vi "氨氮总磷质控流程.vi"(0 "队列输入":refnum<queue>, 5 "氨氮":bool, 7 "氨氮量程切换":enum32{"H", "L", "AUTO"}(ring)=enum."AUTO", 9 "总磷":bool, 11 "总磷量程切换":enum32{"H", "L", "AUTO"}(ring)=enum."AUTO") -> (4 "布尔":bool, 6 "总磷中断报警":bool, 8 "氨氮中断报警":bool)   [LabVIEW 2016]
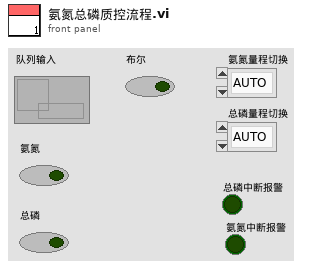
[diagram p1: front panel]
types:
  T1 = enum16{"待机", "启动氨氮水样", "氨氮测量中", "启动氨氮加标", "启动氨氮加标回收", "氨氮加标回收测量中", "启动总磷水样", "总磷水样测量中", "启动总磷加标", "启动总磷加标回收", "总磷加标回收测量中", "结束"}
  T2 = cluster{"站号":u16, "量程切换":enum32{"H", "L", "AUTO"}, "控制命令":enum16{"启动测量", "标样核查", "零点核查", "跨度核查", "空白测试", "平行样测试", "加标回收", "空白校准", "标样校准", "初始化（清洗）", "停止测试", "仪器重启", "校时", "模式设置", "测量间隔设置", "盲样测试"}, "模式设置":enum16{"待机", "连续模式", "周期模式", "定点模式", "受控模式", "手动模式"}, "测量间隔":u16}
  T3 = cluster{"时间标识":timestamp, "设备":string, "日志信息":string}
  T4 = cluster{"系统时间":timestamp, "工作状态":enum16{"空闲", "水样测试", "标样核查", "零点核查", "跨度核查", "空白测试", "平行样测试", "加标回收", "空白校准", "标样校准", "初始化（清洗）"}, "测量模式":enum16{"待机", "连续模式", "周期模式", "定点模式", "受控模式", "手动模式"}, "告警代码":enum16{"无告警", "缺试剂告警", "缺水样告警", "缺蒸馏水告警", "缺标液告警", "仪表漏液告警", "标定异常告警", "超量程告警", "加热异常", "低试剂预警", "超上限告警", "超下限告警", "仪表内部其他异常", "滴定异常告警", "电极异常告警", "量程切换告警", "参数设置告警", "PH电极电位异常", "电导率电极异常", "浊度光度异常", "溶解氧电极异常", "溶解氧光强异常", "温度异常告警", "PH异常告警", "溶解氧异常告警", "电导率异常告警", "浊度异常告警", "叶绿素异常告警", "藻密度异常告警", "蓝绿藻异常告警", "ORP异常告警", "氨氮异常告警", "清洁刷异常告警", "SD卡异常告警", "蓝牙异常告警", "Wifi异常告警", "流程异常告警"}, "故障代码":enum16{"无故障", "电机故障", "温度故障", "通讯故障", "滴定故障"}, "日志代码":u16, "软件版本":u16, "F0":sgl, "F1":sgl, "F2":sgl, "F3":sgl, "T":sgl, "H":sgl, "id":u16, "flowid":u16, "量程":u16, "总磷控温温度1":sgl, "营养盐控温温度2":sgl, "ADC":sgl}
  T5 = enum16{"空闲", "水样测试", "标样核查", "零点核查", "跨度核查", "空白测试", "平行样测试", "加标回收", "空白校准", "标样校准", "初始化（清洗）"}
  T6 = cluster{"因子编码":u32, "单位":u16, "标样参考值":sgl, "水样数据时间":timestamp, "水样实测值":sgl, "水样数据标识":string, "标样数据时间":timestamp, "标样实测值":sgl, "标样数据标识":string, "空白数据时间":timestamp, "空白实测值":sgl, "空白数据标识":string, "零点核查数据时间":timestamp, "零点核查实测值":sgl, "零点核查数据标识":string, "跨度核查数据时间":timestamp, "跨度核查实测值":sgl, "跨度核查数据标识":string, "加标回收数据时间":timestamp, "加标回收实测值":sgl, "加标回收数据标识":string, "平行样数据时间":timestamp, "平行样实测值":sgl, "平行样数据标识":string}
  T7 = cluster{"量程":dbl, "检出限":dbl, "加标前水样浓度":dbl, "加标后水样浓度":dbl, "加标水杯定容体积":dbl, "加标母液浓度":dbl, "加标体积":dbl, "加标回收率":dbl}
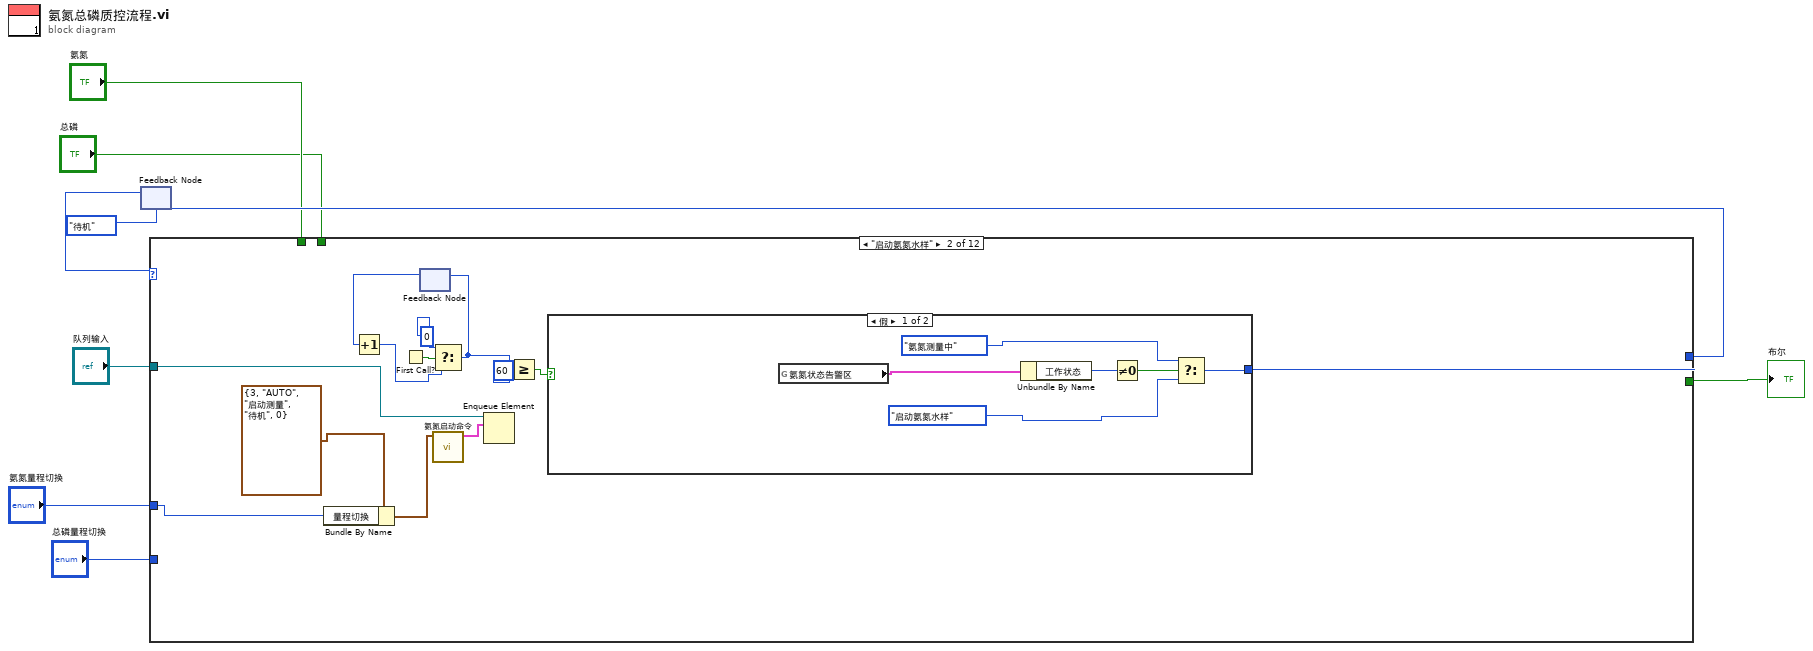
[diagram p0: block diagram]
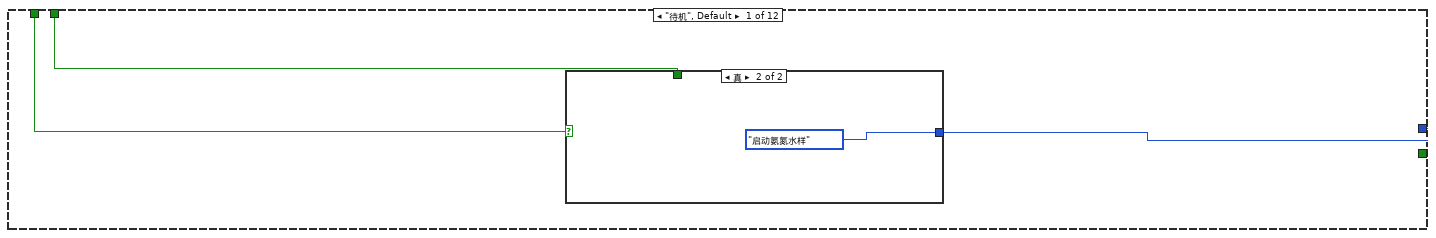
[diagram p2: hidden frame]
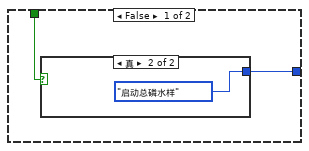
[diagram p3: hidden frame]
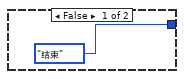
[diagram p4: hidden frame]
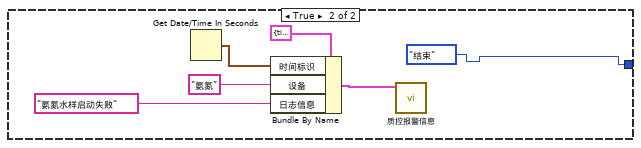
[diagram p5: hidden frame]
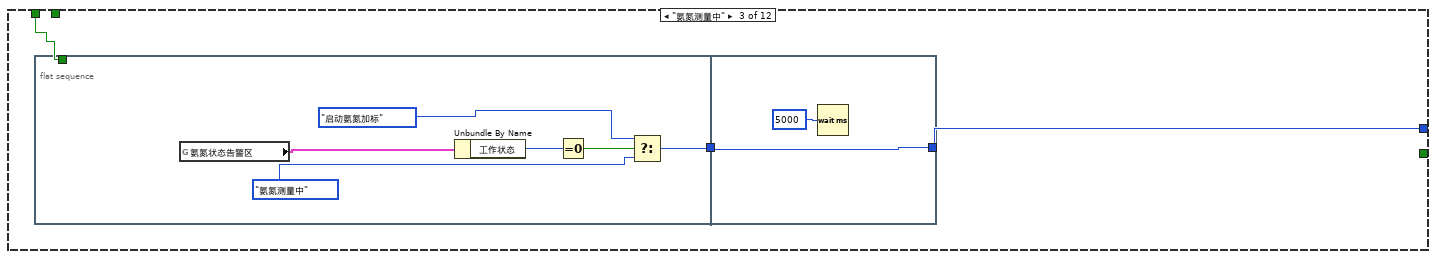
[diagram p6: hidden frame]
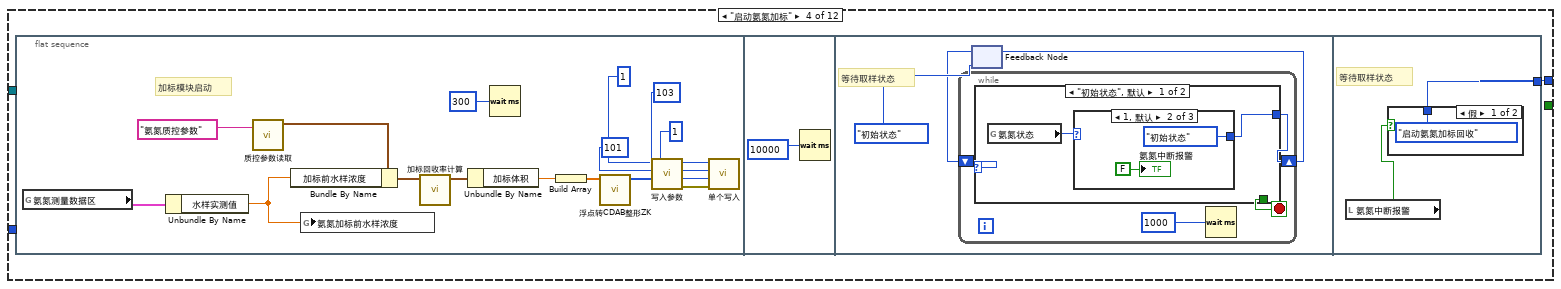
[diagram p7: hidden frame]
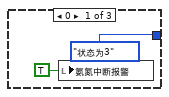
[diagram p8: hidden frame]
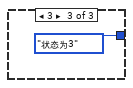
[diagram p9: hidden frame]
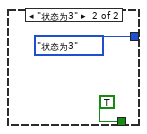
[diagram p10: hidden frame]
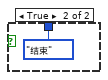
[diagram p11: hidden frame]
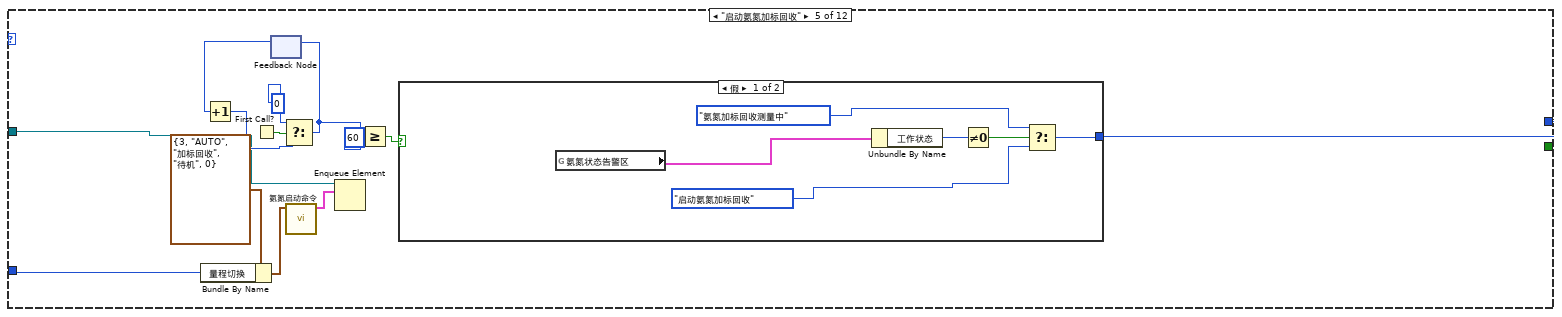
[diagram p12: hidden frame]
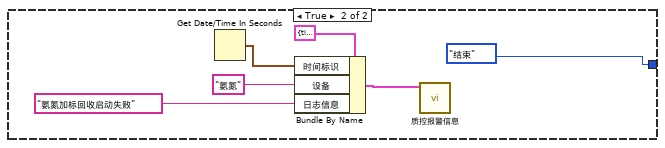
[diagram p13: hidden frame]
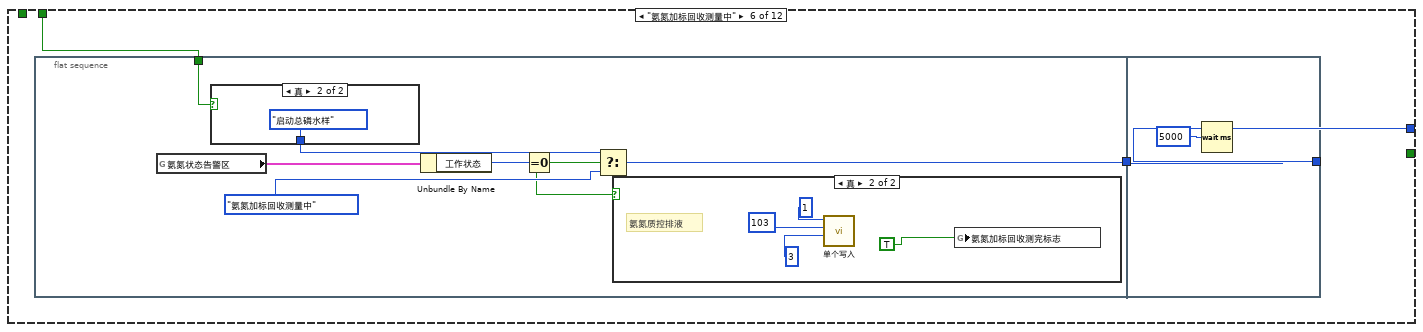
[diagram p14: hidden frame]
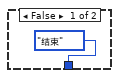
[diagram p15: hidden frame]
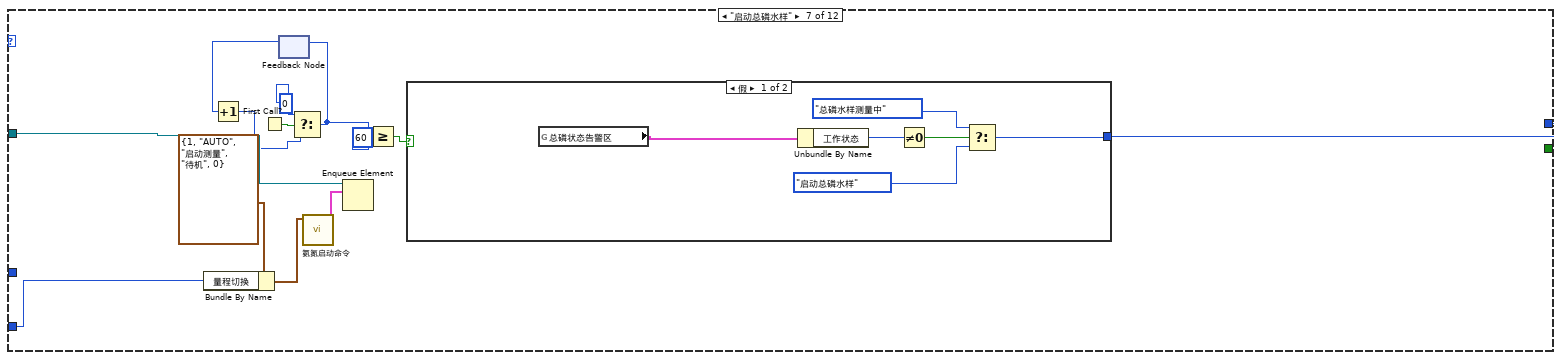
[diagram p17: hidden frame]
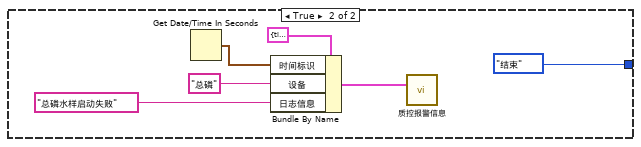
[diagram p18: hidden frame]
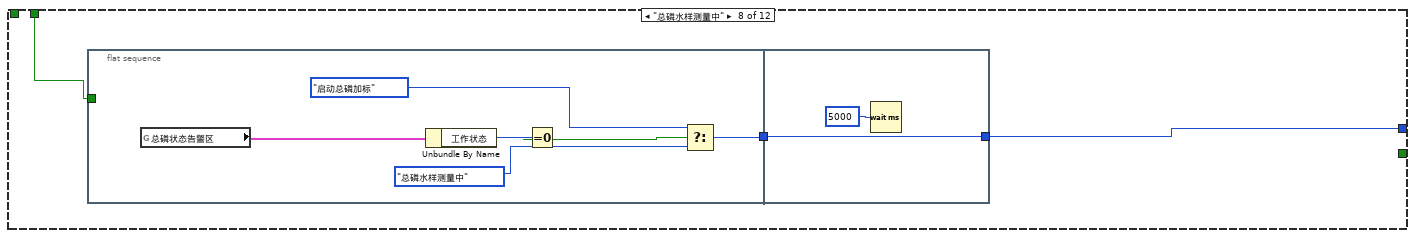
[diagram p19: hidden frame]
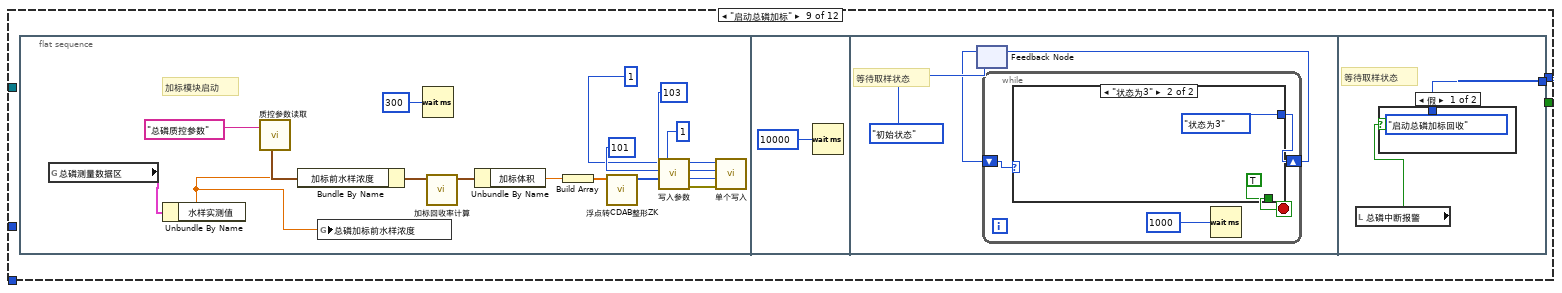
[diagram p20: hidden frame]
diagram:
  n1 = feedback #1(T1."待机") -> (w8:T1)
  n2 = case shown="\"启动氨氮水样\"" w8 {
    tunnel: [w12 w29 w45 w54 w95 w117 w145 w161 w170 w211 w232 T1."结束"] -> w7
    tunnel: "队列输入" -> [_ w30 _ _ w96 _ w146 _ _ w212 _ _]
    tunnel: [_ _ _ _ _ _ _ _ _ _ _ TRUE] -> w4
    tunnel: "总磷" -> [w10 _ _ _ _ w116 _ w159 _ _ _ _]
    tunnel: "氨氮" -> [w11 _ w43 _ _ _ _ _ _ _ _ _]
    tunnel: "氨氮量程切换" -> [_ w19 _ _ w92 _ _ _ _ _ _ _]
    tunnel: "总磷量程切换" -> [_ _ _ _ _ _ w134 _ _ w210 _ _]
    frame "待机", Default {
      n3 = case shown="真" w11 {
        tunnel: [w13 T1."启动氨氮水样"] -> w12
        tunnel: w10 -> [w14 _]
        frame False {
          n4 = case shown="真" w14 {
            tunnel: [T1."结束" T1."启动总磷水样"] -> w13
            frame False {
            }
            frame True {
            }
          }
        }
        frame True {
        }
      }
    }
    frame "启动氨氮水样" {
      n5 = Bundle By Name(cluster=T2 {"站号"=3, "量程切换"=enum."AUTO", "控制命令"=enum."启动测量", "模式设置"=enum."待机", "测量间隔"=0} ("参数"), "量程切换"=w19) -> (w18:T2)
      n6 = First Call?() -> (First Call?: T/F=w27:bool)
      n7 = feedback #2() -> (w26:i32)  [unwired: 1 in]
      n8 = Increment(x=w26) -> (x+1=w25:i32)
      n9 = Select(t=0, s=w27, f=w25) -> (s? t:f=w24:i32)
      n10 = feedback-in #2(w24) -> ()
      n11 = call "氨氮启动命令.vi"("参数"=w18) -> ("启动命令"=w21:cluster{"命令":string, "data":variant})  [unwired: 10 in]
      n12 = Enqueue Element(queue=w30, element=w21) -> ()  [unwired: 2 in, 3 out]
      n13 = Greater Or Equal?(x=w24, y=60) -> (x >= y?=w22:bool)
      n14 = case shown="假" w22 {
        tunnel: [w34 T1."结束"] -> w29
        frame False {
          n15 = global read "与氨氮交互全局.vi" "氨氮状态告警区"() -> (w31:T4)
          n16 = Unbundle By Name(w31) -> ("工作状态"=w36:T5)
          n17 = Not Equal To 0?(x=w36) -> (x != 0?=w35:bool)
          n18 = Select(t=T1."氨氮测量中", s=w35, f=T1."启动氨氮水样") -> (s? t:f=w34:T1)
        }
        frame True {
          n19 = Get Date/Time In Seconds() -> (seconds since 1Jan1904=w42:timestamp)
          n20 = Bundle By Name(cluster=T3 {"时间标识"=timestamp(0 s since 1904-01-01), "设备"="", "日志信息"=""} ("data in"), "时间标识"=w42, "设备"="氨氮", "日志信息"="氨氮水样启动失败") -> (w38:T3)
          n21 = call "质控报警信息.vi"("data in"=w38) -> ()  [unwired: 11 in]
        }
      }
    }
    frame "氨氮测量中" {
      n22 = flat-sequence {
        tunnel: [w50] -> w44
        tunnel: w43 -> [_]
        tunnel: [w53] -> w45
        tunnel: w44 -> [w53]
        frame #0 {
          n23 = global read "与氨氮交互全局.vi" "氨氮状态告警区"() -> (w46:T4)
          n24 = Unbundle By Name(w46) -> ("工作状态"=w51:T5)
          n25 = Equal To 0?(x=w51) -> (x = 0?=w49:bool)
          n26 = Select(t=T1."启动氨氮加标", s=w49, f=T1."氨氮测量中") -> (s? t:f=w50:T1)
        }
        frame #1 {
          n27 = Wait (ms)(milliseconds to wait=u32 5000 ("等待时间（毫秒）")) -> ()  [unwired: 1 out]
        }
      }
    }
    frame "启动氨氮加标" {
      n28 = flat-sequence {
        tunnel: [w88] -> w54
        frame #0 {
          w59 = u16 1 ("value")
          # "加标模块启动"
          n29 = global read "与氨氮交互全局.vi" "氨氮测量数据区"() -> (w56:T6)
          n30 = Unbundle By Name(w56) -> ("水样实测值"=w57:sgl)
          n31 = call "质控参数读取.vi"("section"="氨氮质控参数") -> ("参数"=w67:T7)  [unwired: 9 in, 1 out]
          n32 = Bundle By Name(cluster=w67, "加标前水样浓度"=w57) -> (w68:T7)
          n33 = global write "水样浓度全局.vi" "氨氮加标前水样浓度"(w57) -> ()
          n34 = call "加标回收率计算.vi"("参数"=w68) -> ("参数 out"=w66:T7)  [unwired: 10 in]
          n35 = Unbundle By Name(w66) -> ("加标体积"=w58:dbl)
          n36 = Wait (ms)(milliseconds to wait=u32 300 ("等待时间（毫秒）")) -> ()  [unwired: 1 out]
          n37 = Build Array(w58) -> (w65:dbl[])
          n38 = call "浮点转CDAB整形ZK.vi"("浮点数"=w65) -> ("CDAB整形输出"=w60:u16[])  [unwired: 10 in]
          n39 = call "写入参数.vi"("values"=w60, "starting address"=u16 101, "Slave ID"=w59) -> ("error out"=w64:errorcluster)  [unwired: 8 in]
          n40 = call "单个写入.vi"("Error in"=w64, "value"=u16 1, "address"=u16 103, "Slave ID"=w59) -> ()  [unwired: 7 in, 1 out]
        }
        frame #1 {
          n41 = Wait (ms)(milliseconds to wait=u32 10000 ("等待时间（毫秒）")) -> ()  [unwired: 1 out]
        }
        frame #2 {
          # "等待取样状态"
          n42 = feedback #3(enum16{"初始状态", "状态为3"}."初始状态") -> (w72:enum16{"初始状态", "状态为3"})
          n43 = while {
            shift-right: [w76] -> w71
            shift-left: w72 -> [w77]
            stop <- w75 stop-if-true
            n44 = case shown="\"初始状态\", 默认" w77 {
              tunnel: [w79 enum16{"初始状态", "状态为3"}."状态为3"] -> w76
              tunnel: [_ TRUE] -> w75
              frame "初始状态", Default {
                n45 = global read "加标回收状态全局变量.vi" "氨氮状态"() -> (w78:u16)
                n46 = case shown="1, 默认" w78 {
                  tunnel: [enum16{"初始状态", "状态为3"}."状态为3" enum16{"初始状态", "状态为3"}."初始状态" enum16{"初始状态", "状态为3"}."状态为3"] -> w79
                  frame 0 {
                    n47 = local write "氨氮中断报警"(TRUE ("氨氮中断报警")) -> ()
                  }
                  frame 1, Default {
                    "氨氮中断报警" <- FALSE ("氨氮中断报警")
                  }
                  frame 3 {
                  }
                }
              }
              frame "状态为3" {
              }
            }
            n48 = Wait (ms)(milliseconds to wait=u32 1000 ("等待时间（毫秒）")) -> ()  [unwired: 1 out]
          }
          n49 = feedback-in #3(w71) -> ()
        }
        frame #3 {
          # "等待取样状态"
          n50 = local read "氨氮中断报警"() -> (w87:bool)
          n51 = case shown="假" w87 {
            tunnel: [T1."启动氨氮加标回收" T1."结束"] -> w88
            frame False {
            }
            frame True {
            }
          }
        }
      }
    }
    frame "启动氨氮加标回收" {
      n52 = Bundle By Name(cluster=T2 {"站号"=3, "量程切换"=enum."AUTO", "控制命令"=enum."加标回收", "模式设置"=enum."待机", "测量间隔"=0} ("参数"), "量程切换"=w92) -> (w91:T2)
      n53 = First Call?() -> (First Call?: T/F=w102:bool)
      n54 = feedback #4() -> (w101:i32)  [unwired: 1 in]
      n55 = Increment(x=w101) -> (x+1=w100:i32)
      n56 = Select(t=0, s=w102, f=w100) -> (s? t:f=w99:i32)
      n57 = feedback-in #4(w99) -> ()
      n58 = call "氨氮启动命令.vi"("参数"=w91) -> ("启动命令"=w94:cluster{"命令":string, "data":variant})  [unwired: 10 in]
      n59 = Enqueue Element(queue=w96, element=w94) -> ()  [unwired: 2 in, 3 out]
      n60 = Greater Or Equal?(x=w99, y=60) -> (x >= y?=w97:bool)
      n61 = case shown="假" w97 {
        tunnel: [w107 T1."结束"] -> w95
        frame False {
          n62 = global read "与氨氮交互全局.vi" "氨氮状态告警区"() -> (w104:T4)
          n63 = Unbundle By Name(w104) -> ("工作状态"=w109:T5)
          n64 = Not Equal To 0?(x=w109) -> (x != 0?=w108:bool)
          n65 = Select(t=T1."氨氮加标回收测量中", s=w108, f=T1."启动氨氮加标回收") -> (s? t:f=w107:T1)
        }
        frame True {
          n66 = Get Date/Time In Seconds() -> (seconds since 1Jan1904=w115:timestamp)
          n67 = Bundle By Name(cluster=T3 {"时间标识"=timestamp(0 s since 1904-01-01), "设备"="", "日志信息"=""} ("data in"), "时间标识"=w115, "设备"="氨氮", "日志信息"="氨氮加标回收启动失败") -> (w111:T3)
          n68 = call "质控报警信息.vi"("data in"=w111) -> ()  [unwired: 11 in]
        }
      }
    }
    frame "氨氮加标回收测量中" {
      n69 = flat-sequence {
        tunnel: [w124] -> w118
        tunnel: w116 -> [w120]
        tunnel: [w133] -> w117
        tunnel: w118 -> [w133]
        frame #0 {
          n70 = global read "与氨氮交互全局.vi" "氨氮状态告警区"() -> (w119:T4)
          n71 = case shown="真" w120 {
            tunnel: [T1."结束" T1."启动总磷水样"] -> w122
            frame False {
            }
            frame True {
            }
          }
          n72 = Unbundle By Name(w119) -> ("工作状态"=w125:T5)
          n73 = Equal To 0?(x=w125) -> (x = 0?=w121:bool)
          n74 = Select(t=w122, s=w121, f=T1."氨氮加标回收测量中") -> (s? t:f=w124:T1)
          n75 = case shown="真" w121 {
            frame False {
            }
            frame True {
              # "氨氮质控排液"
              n76 = call "单个写入.vi"("value"=u16 3, "address"=u16 103, "Slave ID"=u8 1) -> ()  [unwired: 8 in, 1 out]
              n77 = global write "质控测完标志全局 1.vi" "氨氮加标回收测完标志"(TRUE) -> ()
            }
          }
        }
        frame #1 {
          n78 = Wait (ms)(milliseconds to wait=u32 5000 ("等待时间（毫秒）")) -> ()  [unwired: 1 out]
        }
      }
    }
    frame "启动总磷水样" {
      n79 = Bundle By Name(cluster=T2 {"站号"=1, "量程切换"=enum."AUTO", "控制命令"=enum."启动测量", "模式设置"=enum."待机", "测量间隔"=0} ("参数"), "量程切换"=w134) -> (w136:T2)
      n80 = First Call?() -> (First Call?: T/F=w143:bool)
      n81 = feedback #5() -> (w142:i32)  [unwired: 1 in]
      n82 = Increment(x=w142) -> (x+1=w141:i32)
      n83 = Select(t=0, s=w143, f=w141) -> (s? t:f=w140:i32)
      n84 = feedback-in #5(w140) -> ()
      n85 = call "氨氮启动命令.vi"("参数"=w136) -> ("启动命令"=w135:cluster{"命令":string, "data":variant})  [unwired: 10 in]
      n86 = Enqueue Element(queue=w146, element=w135) -> ()  [unwired: 2 in, 3 out]
      n87 = Greater Or Equal?(x=w140, y=60) -> (x >= y?=w138:bool)
      n88 = case shown="假" w138 {
        tunnel: [w150 T1."结束"] -> w145
        frame False {
          n89 = global read "与总磷交互全局.vi" "总磷状态告警区"() -> (w147:T4)
          n90 = Unbundle By Name(w147) -> ("工作状态"=w151:T5)
          n91 = Not Equal To 0?(x=w151) -> (x != 0?=w152:bool)
          n92 = Select(t=T1."总磷水样测量中", s=w152, f=T1."启动总磷水样") -> (s? t:f=w150:T1)
        }
        frame True {
          n93 = Get Date/Time In Seconds() -> (seconds since 1Jan1904=w158:timestamp)
          n94 = Bundle By Name(cluster=T3 {"时间标识"=timestamp(0 s since 1904-01-01), "设备"="", "日志信息"=""} ("data in"), "时间标识"=w158, "设备"="总磷", "日志信息"="总磷水样启动失败") -> (w154:T3)
          n95 = call "质控报警信息.vi"("data in"=w154) -> ()  [unwired: 11 in]
        }
      }
    }
    frame "总磷水样测量中" {
      n96 = flat-sequence {
        tunnel: [w166] -> w160
        tunnel: w159 -> [_]
        tunnel: [w169] -> w161
        tunnel: w160 -> [w169]
        frame #0 {
          n97 = global read "与总磷交互全局.vi" "总磷状态告警区"() -> (w162:T4)
          n98 = Unbundle By Name(w162) -> ("工作状态"=w167:T5)
          n99 = Equal To 0?(x=w167) -> (x = 0?=w165:bool)
          n100 = Select(t=T1."启动总磷加标", s=w165, f=T1."总磷水样测量中") -> (s? t:f=w166:T1)
        }
        frame #1 {
          n101 = Wait (ms)(milliseconds to wait=u32 5000 ("等待时间（毫秒）")) -> ()  [unwired: 1 out]
        }
      }
    }
    frame "启动总磷加标" {
      n102 = flat-sequence {
        tunnel: [w204] -> w170
        frame #0 {
          w176 = u16 1 ("value")
          # "加标模块启动"
          n103 = global read "与总磷交互全局.vi" "总磷测量数据区"() -> (w171:T6)
          n104 = Unbundle By Name(w171) -> ("水样实测值"=w173:sgl)
          n105 = call "质控参数读取.vi"("section"="总磷质控参数") -> ("参数"=w174:T7)  [unwired: 9 in, 1 out]
          n106 = Bundle By Name(cluster=w174, "加标前水样浓度"=w173) -> (w184:T7)
          n107 = global write "水样浓度全局.vi" "总磷加标前水样浓度"(w173) -> ()
          n108 = Wait (ms)(milliseconds to wait=u32 300 ("等待时间（毫秒）")) -> ()  [unwired: 1 out]
          n109 = call "加标回收率计算.vi"("参数"=w184) -> ("参数 out"=w183:T7)  [unwired: 10 in]
          n110 = Unbundle By Name(w183) -> ("加标体积"=w175:dbl)
          n111 = Build Array(w175) -> (w182:dbl[])
          n112 = call "浮点转CDAB整形ZK.vi"("浮点数"=w182) -> ("CDAB整形输出"=w177:u16[])  [unwired: 10 in]
          n113 = call "写入参数.vi"("values"=w177, "starting address"=u16 101, "Slave ID"=w176) -> ("error out"=w181:errorcluster)  [unwired: 8 in]
          n114 = call "单个写入.vi"("Error in"=w181, "value"=u16 1, "address"=u16 103, "Slave ID"=w176) -> ()  [unwired: 7 in, 1 out]
        }
        frame #1 {
          n115 = Wait (ms)(milliseconds to wait=u32 10000 ("等待时间（毫秒）")) -> ()  [unwired: 1 out]
        }
        frame #2 {
          # "等待取样状态"
          n116 = feedback #6(enum16{"初始状态", "状态为3"}."初始状态") -> (w188:enum16{"初始状态", "状态为3"})
          n117 = while {
            shift-right: [w192] -> w187
            shift-left: w188 -> [w193]
            stop <- w191 stop-if-true
            n118 = case shown="\"状态为3\"" w193 {
              tunnel: [w195 enum16{"初始状态", "状态为3"}."状态为3"] -> w192
              tunnel: [_ TRUE] -> w191
              frame "初始状态", Default {
                n119 = global read "加标回收状态全局变量.vi" "总磷状态"() -> (w194:u16)
                n120 = case shown="3" w194 {
                  tunnel: [enum16{"初始状态", "状态为3"}."状态为3" enum16{"初始状态", "状态为3"}."初始状态" enum16{"初始状态", "状态为3"}."状态为3"] -> w195
                  frame 0 {
                    n121 = local write "总磷中断报警"(TRUE ("总磷中断报警")) -> ()
                  }
                  frame 1, Default {
                    "总磷中断报警" <- FALSE ("总磷中断报警")
                  }
                  frame 3 {
                  }
                }
              }
              frame "状态为3" {
              }
            }
            n122 = Wait (ms)(milliseconds to wait=u32 1000 ("等待时间（毫秒）")) -> ()  [unwired: 1 out]
          }
          n123 = feedback-in #6(w187) -> ()
        }
        frame #3 {
          # "等待取样状态"
          n124 = local read "总磷中断报警"() -> (w203:bool)
          n125 = case shown="假" w203 {
            tunnel: [T1."启动总磷加标回收" T1."结束"] -> w204
            frame False {
            }
            frame True {
            }
          }
        }
      }
    }
    frame "启动总磷加标回收" {
      n126 = Bundle By Name(cluster=T2 {"站号"=1, "量程切换"=enum."AUTO", "控制命令"=enum."加标回收", "模式设置"=enum."待机", "测量间隔"=0} ("参数"), "量程切换"=w210) -> (w208:T2)
      n127 = First Call?() -> (First Call?: T/F=w218:bool)
      n128 = feedback #7() -> (w217:i32)  [unwired: 1 in]
      n129 = Increment(x=w217) -> (x+1=w216:i32)
      n130 = Select(t=0, s=w218, f=w216) -> (s? t:f=w215:i32)
      n131 = feedback-in #7(w215) -> ()
      n132 = call "氨氮启动命令.vi"("参数"=w208) -> ("启动命令"=w207:cluster{"命令":string, "data":variant})  [unwired: 10 in]
      n133 = Enqueue Element(queue=w212, element=w207) -> ()  [unwired: 2 in, 3 out]
      n134 = Greater Or Equal?(x=w215, y=60) -> (x >= y?=w213:bool)
      n135 = case shown="假" w213 {
        tunnel: [w224 T1."结束"] -> w211
        frame False {
          n136 = global read "与总磷交互全局.vi" "总磷状态告警区"() -> (w221:T4)
          n137 = Unbundle By Name(w221) -> ("工作状态"=w220:T5)
          n138 = Not Equal To 0?(x=w220) -> (x != 0?=w225:bool)
          n139 = Select(t=T1."总磷加标回收测量中", s=w225, f=T1."启动总磷加标回收") -> (s? t:f=w224:T1)
        }
        frame True {
          n140 = Get Date/Time In Seconds() -> (seconds since 1Jan1904=w231:timestamp)
          n141 = Bundle By Name(cluster=T3 {"时间标识"=timestamp(0 s since 1904-01-01), "设备"="", "日志信息"=""} ("data in"), "时间标识"=w231, "设备"="总磷", "日志信息"="总磷启动失败") -> (w227:T3)
          n142 = call "质控报警信息.vi"("data in"=w227) -> ()  [unwired: 11 in]
        }
      }
    }
    frame "总磷加标回收测量中" {
      n143 = flat-sequence {
        tunnel: [w239] -> w233
        tunnel: [w245] -> w232
        tunnel: w233 -> [w245]
        frame #0 {
          n144 = global read "与总磷交互全局.vi" "总磷状态告警区"() -> (w235:T4)
          n145 = Unbundle By Name(w235) -> ("工作状态"=w234:T5)
          n146 = Equal To 0?(x=w234) -> (x = 0?=w236:bool)
          n147 = Select(t=T1."结束", s=w236, f=T1."总磷加标回收测量中") -> (s? t:f=w239:T1)
          n148 = case shown="真" w236 {
            frame False {
            }
            frame True {
              # "总磷质控排液"
              n149 = global write "质控测完标志全局 1.vi" "总磷加标回收测完标志"(TRUE) -> ()
              n150 = call "单个写入.vi"("value"=u16 3, "address"=u16 103, "Slave ID"=u8 1) -> ()  [unwired: 8 in, 1 out]
            }
          }
        }
        frame #1 {
          n151 = Wait (ms)(milliseconds to wait=u32 5000 ("等待时间（毫秒）")) -> ()  [unwired: 1 out]
        }
      }
    }
    frame "结束" {
    }
  }
  "布尔" <- w4
  n152 = feedback-in #1(w7) -> ()
